vi "valves_pumpmanual.vi"(7 "Pump frequency":dbl=15.0 min=1.0 max=100.0, 8 "error in (no error)":errorcluster, 9 "Pumping":refnum<vi>, 10 "Mix pump":refnum<vi>, 11 "COM in":refnum<k24>) -> (0 "error out":errorcluster, 3 "COM out":refnum<k24>)   [LabVIEW 2018]
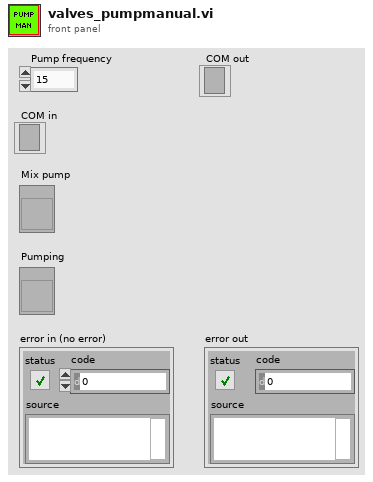
[diagram p1: front panel]
types:
  T1 = cluster{"Step 1":u8[], "Step 2":u8[], "Step 3":u8[], "Step 4":u8[], "Step 5":u8[], "Step 6":u8[]}
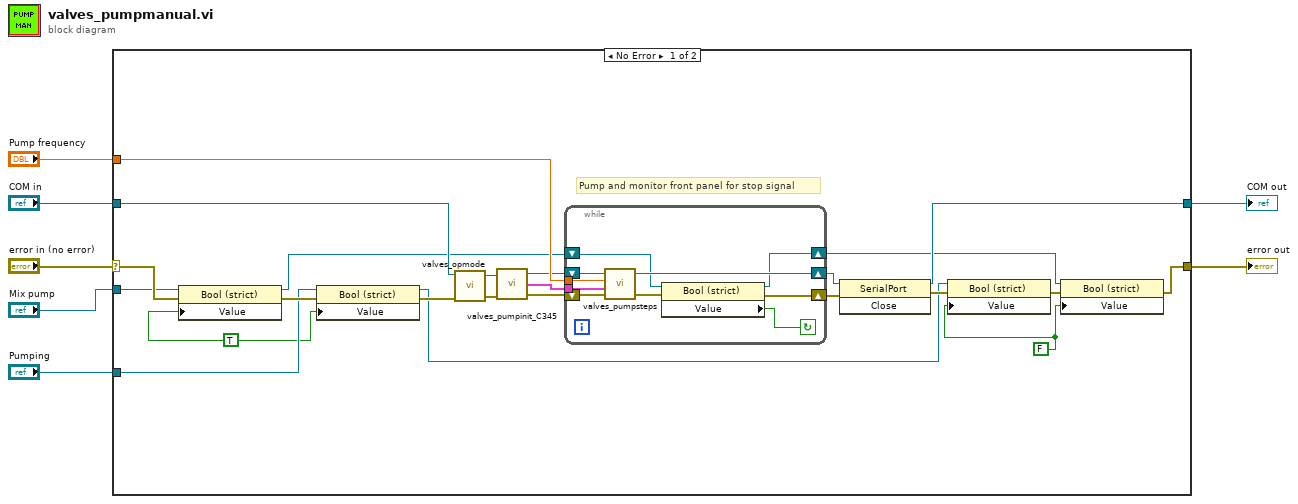
[diagram p0: block diagram]
diagram:
  n1 = case shown="No Error" "error in (no error)" {
    selector: "error in (no error)" -> [w29 w41]
    tunnel: [w30 w41] -> w1
    tunnel: "COM in" -> [w28 w42]
    tunnel: [w27 w42] -> w4
    tunnel: "Pump frequency" -> [w26 _]
    tunnel: "Mix pump" -> [w14 _]
    tunnel: "Pumping" -> [w13 _]
    frame No Error {
      w8 = FALSE
      w12 = TRUE
      # "Pump and monitor front panel for stop signal"
      n2 = property class="Bool (strict)"(reference=w14, error in=w29, "Value"=w12) -> (reference out=w11:refnum<vi>, error out=w20:errorcluster)
      n3 = property class="Bool (strict)"(reference=w13, error in=w20, "Value"=w12) -> (reference out=w9:refnum<vi>, error out=w18:errorcluster)
      n4 = call "valves_opmode.vi"("COM4 in"=w28, "error in"=w18) -> ("COM4 out"=w23:refnum<k24>, "error out"=w25:errorcluster)  [unwired: 5 in]
      n5 = call "valves_pumpinit_C345.vi"("COM4 in"=w23, "error in"=w25) -> ("COM4 out"=w22:refnum<k24>, "Commands out"=w21:T1, "error out"=w24:errorcluster)  [unwired: 3 in]
      n6 = while {
        tunnel: w21 -> [w38]
        shift-right: [w37] -> w15
        shift-left: w22 -> [w39]
        tunnel: w26 -> [w36]
        shift-right: [w34] -> w17
        shift-left: w24 -> [w40]
        shift-right: [w32] -> w10
        shift-left: w11 -> [w33]
        stop <- w31 continue-if-true
        n7 = call "valves_pumpsteps.vi"("COM4 in"=w39, "Pump frequency"=w36, "Commands in"=w38, "error in"=w40) -> ("COM4 out"=w37:refnum<k24>, "error out"=w35:errorcluster)  [unwired: 3 in]
        n8 = property class="Bool (strict)"(reference=w33, error in=w35) -> (reference out=w32:refnum<vi>, error out=w34:errorcluster, "Value"=w31:bool)
      }
      n9 = invoke class="SerialPort" method="Close"(reference=w15, error in=w17) -> (reference out=w27:refnum<k24>, error out=w16:errorcluster)  [unwired: 1 in, 1 out]
      n10 = property class="Bool (strict)"(reference=w9, error in=w16, "Value"=w8) -> (error out=w19:errorcluster)  [unwired: 1 out]
      n11 = property class="Bool (strict)"(reference=w10, error in=w19, "Value"=w8) -> (error out=w30:errorcluster)  [unwired: 1 out]
    }
    frame Error {
    }
  }
  "error out" <- w1
  "COM out" <- w4
